vi "CollectData.vi"(5 "VISA resource name":refnum<visa-resource-name>="COM1" caption="VISA资源名称", 6 "mbfUartClearOne":bool=TRUE, 8 "写指令":bool=TRUE) -> (0 "波形图表":i32(graph), 1 "命令":string, 2 "Time":u32, 3 "缓冲区数据":u32, 4 "Result":string[](array[string]), 7 "mbfDealData":bool, 9 "mu08SendCmd":u8)   [LabVIEW 2011]
uses:
  <vilib>/Instr/_visa.llb/VISA Configure Serial Port (Instr).vi
panel:
  out "mu08ArrayBuf0":u8[](array[numeric]) format="0x%x"
  out "mu08BufSize":u8
  out "mu16ArrayBuf0":u16
  out "mu08ArrayDatas":u8[](array[numeric]) format="0x%x"
  out "mu08ArrayDatasSize":u16
  in  "CmdNumCount":u8
  # "WW专用   数据总数为 278"
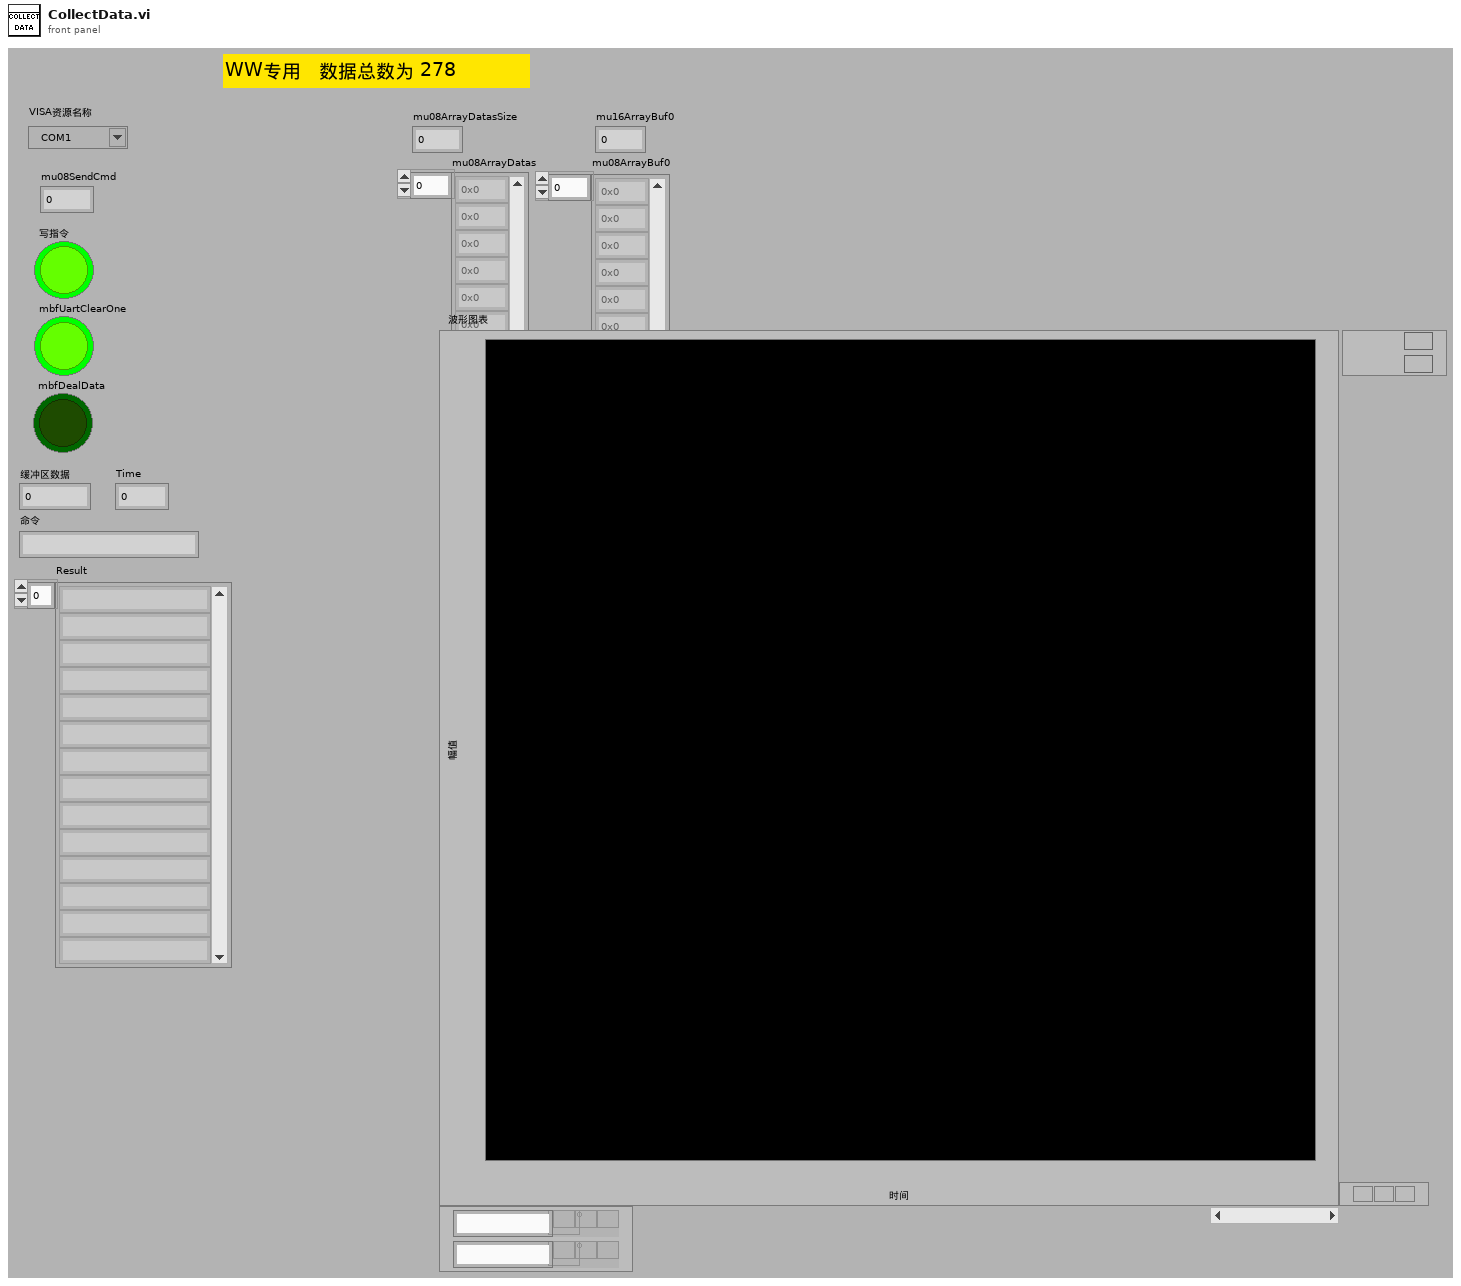
[diagram p1: front panel]
types:
  T1 = enum16{"open", "replace", "create", "open or create", "replace or create", "replace or create with confirmation"}
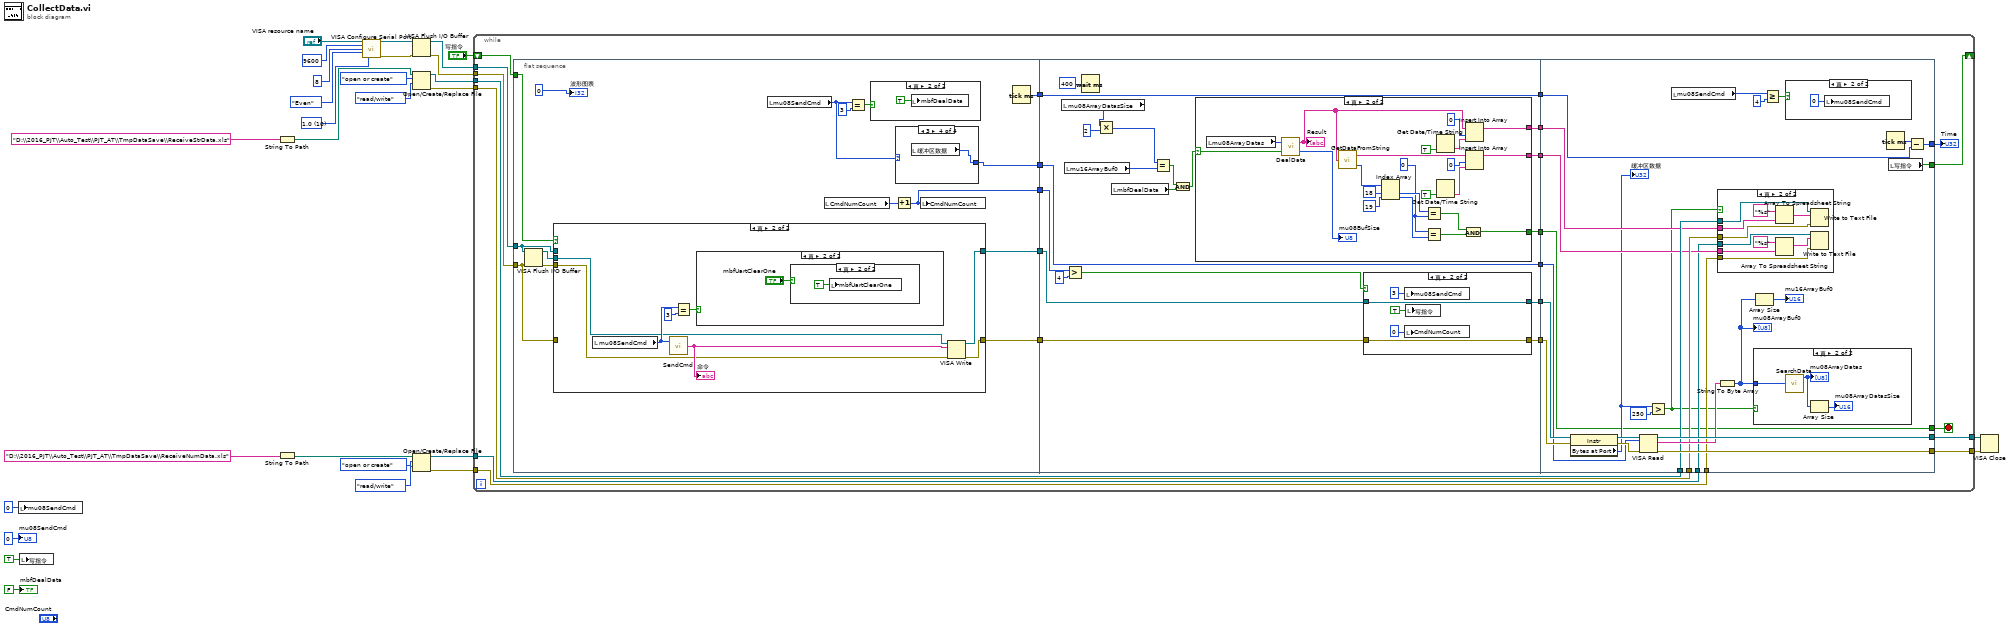
[diagram p0: block diagram]
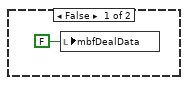
[diagram p2: hidden frame]
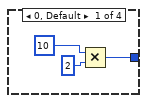
[diagram p3: hidden frame]
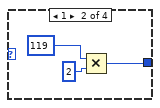
[diagram p4: hidden frame]
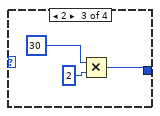
[diagram p5: hidden frame]
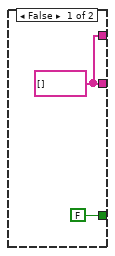
[diagram p9: hidden frame]
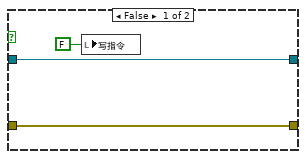
[diagram p10: hidden frame]
diagram:
  w24 = u16 10 items=["1.0"=10, "1.5"=15, "2.0"=20] ("stop bits (10: 1 bit)")
  n1 = local write "mu08SendCmd"(u8 0 ("Cmd值")) -> ()
  n2 = local write "写指令"(TRUE ("写指令")) -> ()
  n3 = String To Path(string="D:\\2016_PJT\\Auto_Test\\PJT_AT\\TmpDataSave\\ReceiveStrData.xls") -> (path=w10:path)
  n4 = String To Path(string="D:\\2016_PJT\\Auto_Test\\PJT_AT\\TmpDataSave\\ReceiveNumData.xls") -> (path=w2:path)
  n5 = call-poly "VISA Configure Serial Port"("VISA resource name"="VISA resource name", "baud rate (9600)"=u32 9600, "data bits (8)"=u16 8, "parity (0:none)"=enum16{"None", "Odd", "Even", "Mark", "Space"}."Even", "stop bits (10: 1 bit)"=w24) -> ("VISA resource name out"=w20:refnum<visa-resource-name>, "error out"=w19:errorcluster)  [unwired: 9 in]
  n6 = VISA Flush I/O Buffer(VISA resource name=w20, error in (no error)=w19) -> (VISA resource name out=w18:refnum<visa-resource-name>, error out=w17:errorcluster)  [unwired: 1 in]
  n7 = Open/Create/Replace File(file path (use dialog)=w10, operation (0:open)=T1."open or create" ("操作(0:open)"), access (0:read/write)=enum16{"read/write", "read-only", "write-only"}."read/write" ("权限(0:read/write)")) -> (refnum out=w9:refnum<file>, error out=w8:errorcluster)  [unwired: 3 in, 1 out]
  n8 = Open/Create/Replace File(file path (use dialog)=w2, operation (0:open)=T1."open or create" ("操作(0:open)"), access (0:read/write)=enum16{"read/write", "read-only", "write-only"}."read/write" ("权限(0:read/write)")) -> (refnum out=w6:refnum<file>, error out=w7:errorcluster)  [unwired: 3 in, 1 out]
  n9 = while {
    tunnel: w18 -> [w52]
    tunnel: w17 -> [w51]
    tunnel: [w48] -> w23
    tunnel: [w47] -> w22
    shift-right: [w45] -> _
    shift-left: "写指令" -> [w46]
    tunnel: w9 -> [w39]
    tunnel: w8 -> [w38]
    tunnel: w7 -> [w32]
    tunnel: w6 -> [w31]
    stop <- w29 stop-if-true
    n10 = flat-sequence {
      tunnel: w52 -> [w59]
      tunnel: w51 -> [w58]
      tunnel: [w67] -> w50
      tunnel: [w66] -> w49
      tunnel: w46 -> [w65]
      tunnel: [w63] -> w44
      tunnel: [w53] -> w40
      tunnel: [w55] -> w36
      tunnel: w50 -> [w105]
      tunnel: w49 -> [w104]
      tunnel: w44 -> [w108]
      tunnel: [w107] -> w43
      tunnel: [w106] -> w42
      tunnel: [w103] -> w41
      tunnel: w40 -> [w103]
      tunnel: [w102] -> w37
      tunnel: w36 -> [w101]
      tunnel: [w101] -> w35
      tunnel: [w100] -> w33
      tunnel: [w95] -> w30
      tunnel: w43 -> [w165]
      tunnel: w42 -> [w164]
      tunnel: w41 -> [w160]
      tunnel: [w168] -> w48
      tunnel: [w167] -> w47
      tunnel: [w159] -> w45
      tunnel: w39 -> [w157]
      tunnel: w38 -> [w156]
      tunnel: w37 -> [w155]
      tunnel: w35 -> [w153]
      tunnel: [w152] -> w34
      tunnel: w33 -> [w151]
      tunnel: w32 -> [w150]
      tunnel: w31 -> [w149]
      tunnel: [w144] -> w29
      tunnel: w30 -> [w144]
      frame #0 {
        n11 = VISA Flush I/O Buffer(VISA resource name=w59, error in (no error)=w58) -> (VISA resource name out=w56:refnum<visa-resource-name>, error out=w57:errorcluster)  [unwired: 1 in]
        n12 = case shown="真" w65 {
          tunnel: w59 -> [w81 _]
          tunnel: w58 -> [w80 _]
          tunnel: [w81 w89] -> w67
          tunnel: [w80 w88] -> w66
          tunnel: w57 -> [_ w83]
          tunnel: w56 -> [_ w82]
          frame False {
          }
          frame True {
            n13 = local read "mu08SendCmd"() -> (w85:u8)
            n14 = call "SendCmd.vi"("索引 (行)"=w85) -> ("字符串"=w87:string)  [unwired: 1 in]
            "命令" <- w87
            n15 = Equal?(x=w85, y=u8 3) -> (x = y?=w84:bool)
            n16 = case shown="真" w84 {
              frame False {
              }
              frame True {
                n17 = case shown="真" "mbfUartClearOne" {
                  frame False {
                  }
                  frame True {
                    n18 = local write "mbfUartClearOne"(TRUE ("mbfUartClearOne")) -> ()
                  }
                }
              }
            }
            n19 = VISA Write(VISA resource name=w82, write buffer=w87, error in (no error)=w83) -> (VISA resource name out=w89:refnum<visa-resource-name>, error out=w88:errorcluster)  [unwired: 1 out]
          }
        }
        n20 = local read "mu08SendCmd"() -> (w62:u8)
        n21 = local read "CmdNumCount"() -> (w64:u8)
        n22 = Equal?(x=w62, y=u8 3) -> (x = y?=w60:bool)
        n23 = case shown="真" w60 {
          frame False {
            n24 = local write "mbfDealData"(FALSE ("mbfDealData")) -> ()
          }
          frame True {
            n25 = local write "mbfDealData"(TRUE ("mbfDealData")) -> ()
          }
        }
        n26 = case shown="3" w62 {
          tunnel: [w70 w73 w76 w79] -> w53
          frame 0, Default {
            n27 = Multiply(x=10, y=2) -> (x*y=w70:i32)
          }
          frame 1 {
            n28 = Multiply(x=119, y=2) -> (x*y=w73:i32)
          }
          frame 2 {
            n29 = Multiply(x=30, y=2) -> (x*y=w76:i32)
          }
          frame 3 {
            n30 = local read "缓冲区数据"() -> (w79:u32)
          }
        }
        n31 = Increment(x=w64) -> (x+1=w63:u8)
        n32 = local write "CmdNumCount"(w63) -> ()
        n33 = Tick Count (ms)() -> (millisecond timer value=w55:u32)
        "波形图表" <- 0
      }
      frame #1 {
        n34 = local read "mu08ArrayDatasSize"() -> (w94:u16)
        n35 = local read "mu16ArrayBuf0"() -> (w99:u16)
        n36 = Greater?(x=w108, y=u8 4) -> (0:w109:bool)
        n37 = Wait (ms)(milliseconds to wait=u32 400 ("等待时间（毫秒）")) -> ()  [unwired: 1 out]
        n38 = Multiply(x=w94, y=u8 2) -> (x*y=w92:u16)
        n39 = local read "mbfDealData"() -> (w98:bool)
        n40 = Equal?(x=w92, y=w99) -> (x = y?=w97:bool)
        n41 = And(x=w97, y=w98) -> (x .and. y?=w96:bool)
        n42 = case shown="真" w96 {
          selector: w96 -> [_ w114]
          tunnel: [w113 w132] -> w102
          tunnel: [w113 w126] -> w100
          tunnel: [FALSE w116] -> w95
          frame False {
            w113 = string[] []
          }
          frame True {
            w120 = u32 0 ("y")
            n43 = local read "mu08ArrayDatas"() -> (w115:u8[])
            n44 = call "DealData.vi"("mbfDealData"=w114, "ArrayIn"=w115) -> ("mu08BufSize"=→"mu08BufSize":u8, "Result"=w130:string[])
            "Result" <- w130
            n45 = call "GetDataFromString.vi"("strArrayIn"=w130) -> ("strArrayBuf"=w125:string[], "mu32ArrayOut"=w124:u32[])
            n46 = Index Array(array=w124, index #1=18 ("索引"), index #2=19 ("索引")) -> (element #1=w121:u32, element #2=w119:u32)
            n47 = Equal?(x=w121, y=w120) -> (x = y?=w118:bool)
            n48 = Equal?(x=w120, y=w119) -> (x = y?=w117:bool)
            n49 = Get Date/Time String(want seconds? (F)=TRUE ("需要秒？(F)")) -> (time string=w133:string)  [unwired: 2 in, 1 out]
            n50 = Get Date/Time String(want seconds? (F)=TRUE ("需要秒？(F)")) -> (time string=w128:string)  [unwired: 2 in, 1 out]
            n51 = And(x=w118, y=w117) -> (x .and. y?=w116:bool)
            n52 = Insert Into Array(array=w130, index=0 ("索引"), new element=w133) -> (w132:string[])
            n53 = Insert Into Array(array=w125, index=0 ("索引"), new element=w128) -> (w126:string[])
          }
        }
        n54 = case shown="真" w109 {
          tunnel: [w137 w141] -> w107
          tunnel: [w136 w140] -> w106
          tunnel: w105 -> [w137 w141]
          tunnel: w104 -> [w136 w140]
          frame False {
            n55 = local write "写指令"(FALSE ("写指令")) -> ()
          }
          frame True {
            n56 = local write "mu08SendCmd"(u8 3 ("mu08SendCmd")) -> ()
            n57 = local write "CmdNumCount"(u8 0 ("CmdNumCount")) -> ()
            n58 = local write "写指令"(TRUE ("写指令")) -> ()
          }
        }
      }
      frame #2 {
        n59 = property class="Instr"(reference=w165, error in=w164) -> (reference out=w170:refnum<visa-resource-name>, error out=w169:errorcluster, "Bytes at Port"=w147:u32)
        "缓冲区数据" <- w147
        n60 = VISA Read(VISA resource name=w170, byte count=w160, error in (no error)=w169) -> (VISA resource name out=w168:refnum<visa-resource-name>, read buffer=w166:string, error out=w167:errorcluster)  [unwired: 1 out]
        n61 = Greater?(x=w147, y=250) -> (0:w146:bool)
        n62 = local read "mu08SendCmd"() -> (w163:u8)
        n63 = case shown="真" w146 {
          tunnel: w157 -> [_ w181]
          tunnel: w156 -> [_ w180]
          tunnel: w155 -> [_ w179]
          tunnel: w151 -> [_ w178]
          tunnel: w150 -> [_ w175]
          tunnel: w149 -> [_ w174]
          frame False {
          }
          frame True {
            n64 = Array To Spreadsheet String(array=w179, 3:"%s" ("格式字符串")) -> (spreadsheet string=w183:string)  [unwired: 1 in]
            n65 = Array To Spreadsheet String(array=w178, 3:"%s" ("格式字符串")) -> (spreadsheet string=w176:string)  [unwired: 1 in]
            n66 = Write to Text File(file (use dialog)=w181, text=w183, error in=w180) -> ()  [unwired: 1 in, 3 out]
            n67 = Write to Text File(file (use dialog)=w174, text=w176, error in=w175) -> ()  [unwired: 1 in, 3 out]
          }
        }
        n68 = String To Byte Array(string=w166) -> (unsigned byte array=w145:u8[])
        "mu08ArrayBuf0" <- w145
        n69 = case shown="真" w146 {
          tunnel: w145 -> [_ w172]
          frame False {
          }
          frame True {
            n70 = call "SearchData.vi"("ArrayIn"=w172) -> ("ArrayOut"=w171:u8[])  [unwired: 2 out]
            "mu08ArrayDatas" <- w171
            n71 = Array Size(array=w171) -> (size(s)=→"mu08ArrayDatasSize":i32)
          }
        }
        n72 = Array Size(array=w145) -> (size(s)=→"mu16ArrayBuf0":i32)
        n73 = Greater Or Equal?(x=w163, y=u8 4) -> (x >= y?=w161:bool)
        n74 = case shown="真" w161 {
          frame False {
          }
          frame True {
            n75 = local write "mu08SendCmd"(u8 0 ("Cmd值")) -> ()
          }
        }
        n76 = Tick Count (ms)() -> (millisecond timer value=w154:u32)
        n77 = local read "写指令"() -> (w159:bool)
        n78 = Subtract(x=w154, y=w153) -> (x-y=w152:u32)
      }
    }
    "Time" <- w34
  }
  n79 = VISA Close(VISA resource name=w23, error in (no error)=w22) -> ()  [unwired: 1 out]
  "mu08SendCmd" <- u8 0 ("mu08SendCmd")
  "mbfDealData" <- FALSE ("mbfDealData")
